vi "FPGAReadWrite.vi"(7 "Enum":enum16{"WRITE_DIO", "WRITE_AO", "READ_AI"}(ring), 8 "error in":errorcluster, 10 "AO cluster":T2, 11 "DIOcluster":T1) -> (0 "error out":errorcluster, 3 "AI Cluster":T3)   [LabVIEW 2019]
uses:
  <vilib>/Utility/error.llb/Error Cluster From Error Code.vi
  <vilib>/rvi/errors/niLvFpgaAdjustHostInterfaceError.vi
  <vilib>/rvi/interface/nirviReadWriteControl/nirviReadWriteControl.xnode
  NiFpgaLv.dll
  <vilib>/rvi/interface/Simulation/niFpgaSimulationCallBeginRW.vi
panel:
  # "MW7"
  # "MW8"
  # "XM"
  # "RF"
  # "XR"
  # "AOM"
  # "EOM"
  # "MW"
  # "MW1"
  # "MW2"
  # "MW3"
  # "MW4"
  # "MW5"
  # "MW6"
  # "AOM"
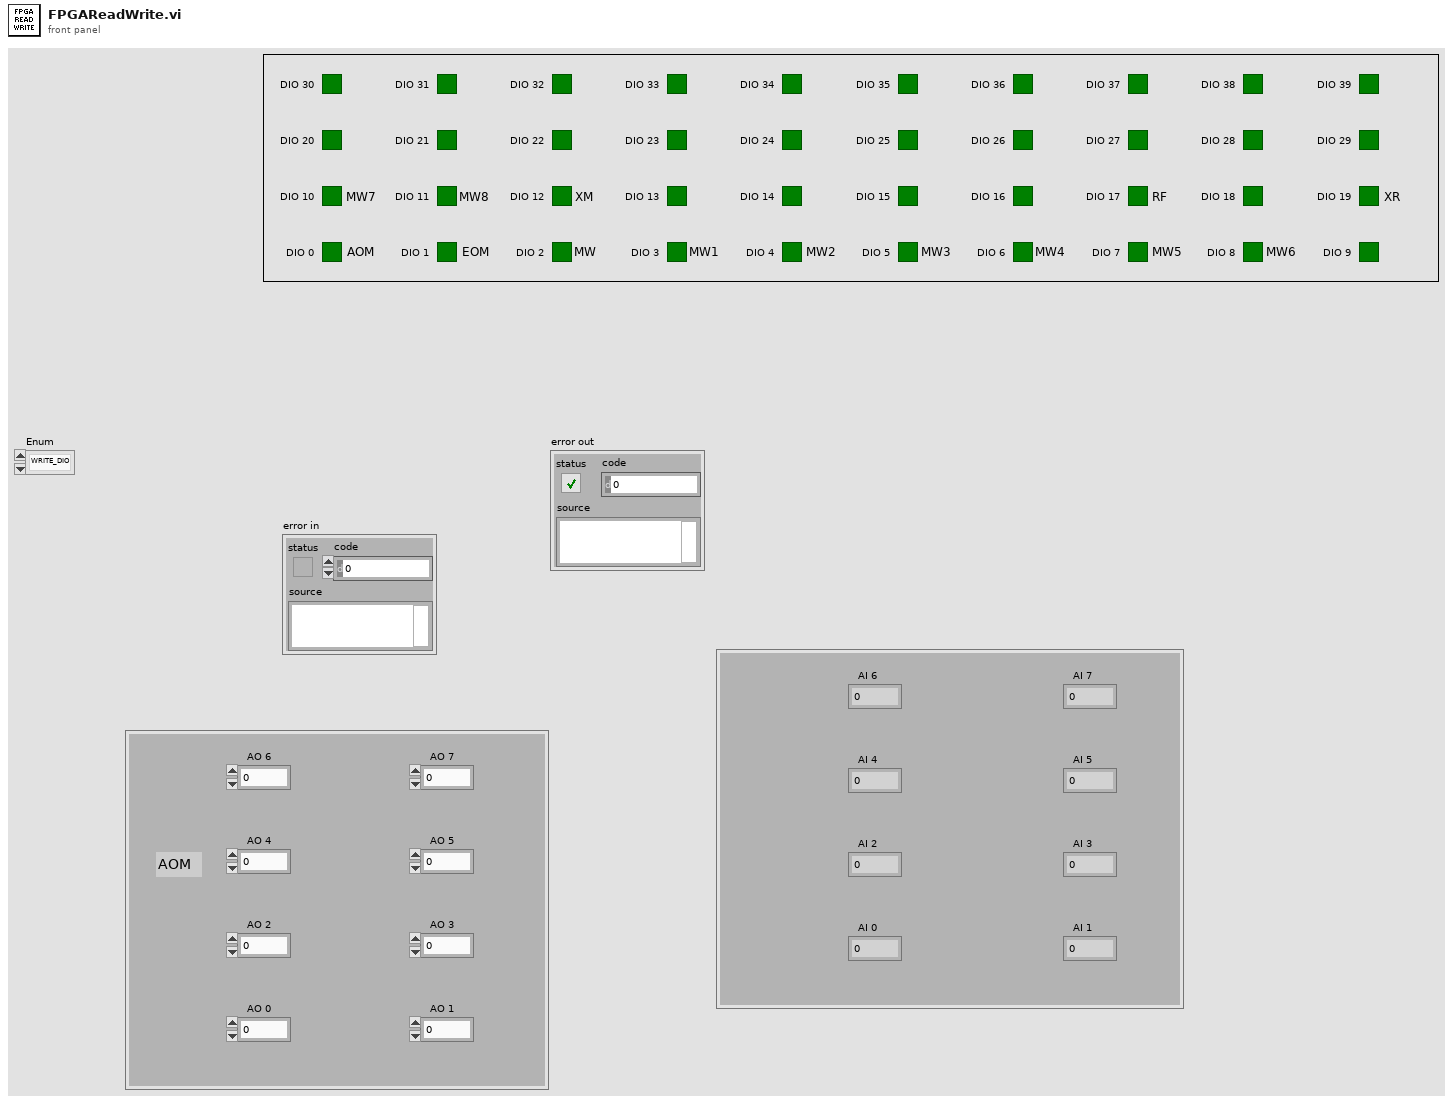
[diagram p1: front panel]
types:
  T1 = cluster{"DIO 0":bool, "DIO 1":bool, "DIO 2":bool, "DIO 3":bool, "DIO 4":bool, "DIO 5":bool, "DIO 6":bool, "DIO 7":bool, "DIO 8":bool, "DIO 9":bool, "DIO 10":bool, "DIO 11":bool, "DIO 12":bool, "DIO 13":bool, "DIO 14":bool, "DIO 15":bool, "DIO 16":bool, "DIO 17":bool, "DIO 18":bool, "DIO 19":bool, "DIO 20":bool, "DIO 21":bool, "DIO 22":bool, "DIO 23":bool, "DIO 24":bool, "DIO 25":bool, "DIO 26":bool, "DIO 27":bool, "DIO 28":bool, "DIO 29":bool, "DIO 30":bool, "DIO 31":bool, "DIO 32":bool, "DIO 33":bool, "DIO 34":bool, "DIO 35":bool, "DIO 36":bool, "DIO 37":bool, "DIO 38":bool, "DIO 39":bool}
  T2 = cluster{"AO 0":dbl, "AO 1":dbl, "AO 2":dbl, "AO 3":dbl, "AO 4":dbl, "AO 5":dbl, "AO 6":dbl, "AO 7":dbl}
  T3 = cluster{"AI 0":dbl, "AI 1":dbl, "AI 2":dbl, "AI 3":dbl, "AI 4":dbl, "AI 5":dbl, "AI 6":dbl, "AI 7":dbl}
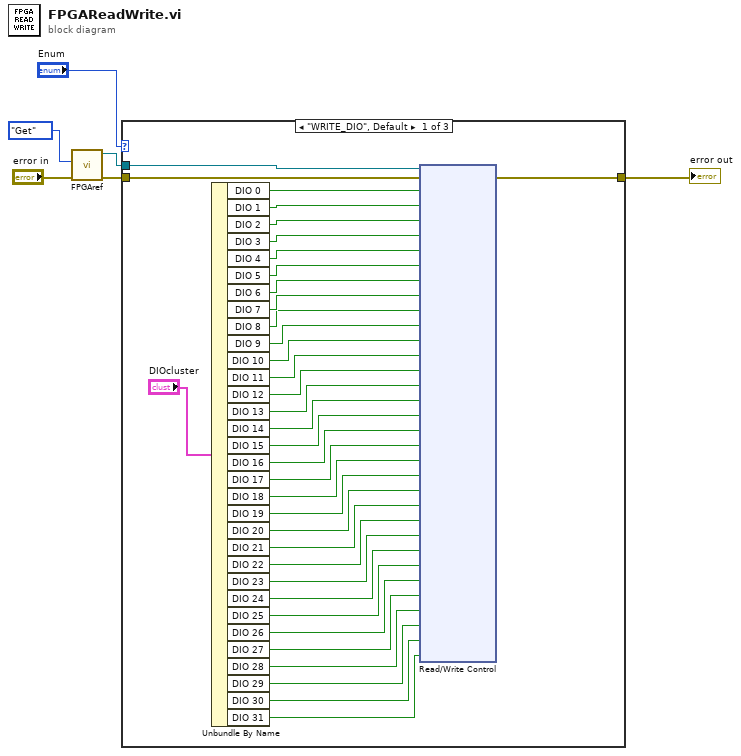
[diagram p0: block diagram]
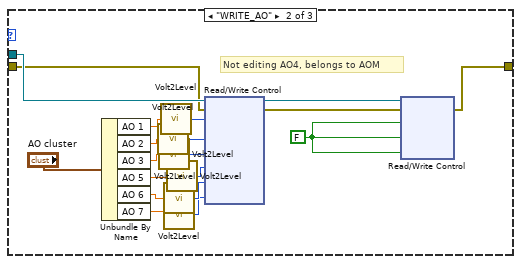
[diagram p2: hidden frame]
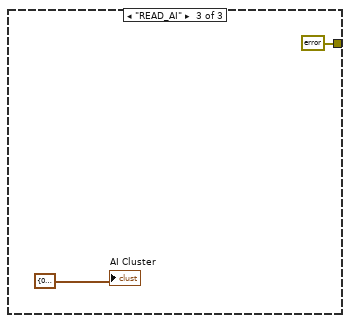
[diagram p3: hidden frame]
diagram:
  n1 = call "FPGAref.vi"("error in"="error in", "Enum"=enum16{"Set", "Get"}."Get") -> ("error out"=w2:errorcluster, "FPGA VI Reference Out 2"=w3:refnum<k20>)  [unwired: 4 in]
  n2 = case shown="\"WRITE_DIO\", Default" "Enum" {
    tunnel: w3 -> [w10 w45 _]
    tunnel: w2 -> [w9 w44 _]
    tunnel: [w8 w43 errorcluster {"status"=FALSE, "code"=0, "source"=""} ("error out")] -> w1
    frame "WRITE_DIO", Default {
      n3 = Unbundle By Name("DIOcluster") -> ("DIO 0"=w42:bool, "DIO 1"=w41:bool, "DIO 2"=w40:bool, "DIO 3"=w39:bool, "DIO 4"=w38:bool, "DIO 5"=w37:bool, "DIO 6"=w36:bool, "DIO 7"=w35:bool, "DIO 8"=w34:bool, "DIO 9"=w33:bool, "DIO 10"=w32:bool, "DIO 11"=w31:bool, "DIO 12"=w30:bool, "DIO 13"=w29:bool, "DIO 14"=w28:bool, "DIO 15"=w27:bool, "DIO 16"=w26:bool, "DIO 17"=w25:bool, "DIO 18"=w24:bool, "DIO 19"=w23:bool, "DIO 20"=w22:bool, "DIO 21"=w21:bool, "DIO 22"=w20:bool, "DIO 23"=w19:bool, "DIO 24"=w18:bool, "DIO 25"=w17:bool, "DIO 26"=w16:bool, "DIO 27"=w15:bool, "DIO 28"=w14:bool, "DIO 29"=w13:bool, "DIO 30"=w12:bool, "DIO 31"=w11:bool)
      n4 = xnode "Read/Write Control"("FPGA VI Reference In"=w10, "error in"=w9, "AOM"=w42, "EOM"=w41, "Microwave"=w40, "dds/ag"=w39, "DIO4"=w38, "DIO5"=w37, "DIO6"=w36, "DIO7"=w35, "DIO8"=w34, "DIO9"=w33, "DIO10"=w32, "DIO11"=w31, "D12"=w30, "D13"=w29, "D14"=w28, "D15"=w27, "D16"=w26, "D17"=w25, "D18"=w24, "D19"=w23, "D20"=w22, "D21"=w21, "D22"=w20, "D23"=w19, "D24"=w18, "D25"=w17, "D26"=w16, "D27"=w15, "D28"=w14, "D29"=w13, "D30"=w12, "D31"=w11) -> ("error out"=w8:errorcluster)  [unwired: 1 out]
    }
    frame "WRITE_AO" {
      w59 = FALSE ("AO1")
      # "Not editing AO4, belongs to AOM"
      n5 = Unbundle By Name("AO cluster") -> ("AO 1"=w57:dbl, "AO 2"=w55:dbl, "AO 3"=w54:dbl, "AO 5"=w53:dbl, "AO 6"=w52:dbl, "AO 7"=w51:dbl)
      n6 = call "Volt2Level.vi"("voltage /V"=w55) -> ("level"=w50:i16)
      n7 = call "Volt2Level.vi"("voltage /V"=w54) -> ("level"=w49:i16)
      n8 = call "Volt2Level.vi"("voltage /V"=w57) -> ("level"=w56:i16)
      n9 = call "Volt2Level.vi"("voltage /V"=w52) -> ("level"=w47:i16)
      n10 = call "Volt2Level.vi"("voltage /V"=w51) -> ("level"=w46:i16)
      n11 = call "Volt2Level.vi"("voltage /V"=w53) -> ("level"=w48:i16)
      n12 = xnode "Read/Write Control"("FPGA VI Reference In"=w45, "error in"=w44, "AO1 off"=w56, "AO2 off"=w50, "AO3 off"=w49, "AO5"=w48, "AO6"=w47, "AO7"=w46) -> ("FPGA VI Reference Out"=w61:refnum<k20>, "error out"=w60:errorcluster)
      n13 = xnode "Read/Write Control"("FPGA VI Reference In"=w61, "error in"=w60, "AO1"=w59, "AO2"=w59, "AO3"=w59) -> ("error out"=w43:errorcluster)  [unwired: 1 out]
    }
    frame "READ_AI" {
      "AI Cluster" <- T3 {"AI 0"=0.0, "AI 1"=0.0, "AI 2"=0.0, "AI 3"=0.0, "AI 4"=0.0, "AI 5"=0.0, "AI 6"=0.0, "AI 7"=0.0} ("AI Cluster")
    }
  }
  "error out" <- w1
